vi "Get All Matched Nodes.vi"(8 "error in (no error)":errorcluster, 10 "XPath expression":string, 11 "node in":refnum<k20>) -> (0 "error out":errorcluster, 2 "node result array":refnum<k20>[](array[refnum]), 3 "node out":refnum<k20>)   [LabVIEW 2020, in "NI_XML.lvlib"]
doc: "Returns all the nodes within <B>node in</B> that match the <B>XPath expression</B>."
uses:
  <vilib>/xml/NI_XML.lvlib
  DOMUserDefRef.dll
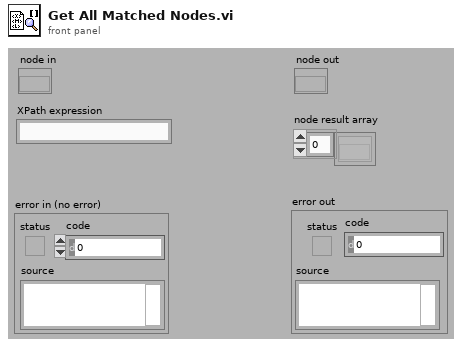
[diagram p1: front panel]
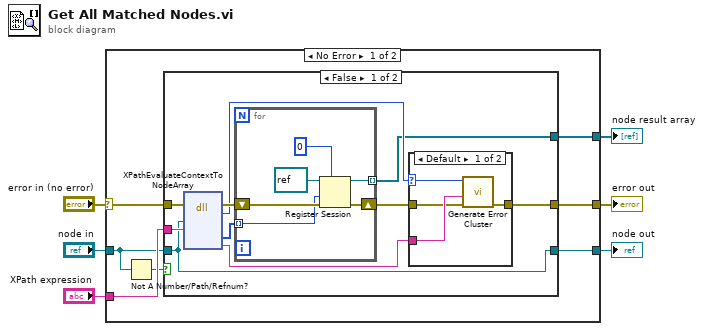
[diagram p0: block diagram]
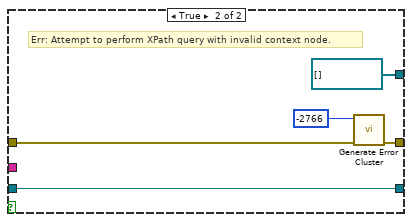
[diagram p3: hidden frame]
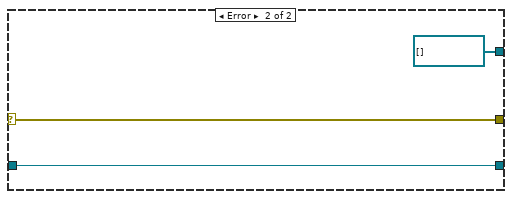
[diagram p4: hidden frame]
diagram:
  n1 = case shown="No Error" "error in (no error)" {
    selector: "error in (no error)" -> [w7 w42]
    tunnel: "XPath expression" -> [w13 _]
    tunnel: [w12 w42] -> w5
    tunnel: [w11 refnum<k20>[] []] -> w4
    tunnel: [w10 w41] -> w3
    tunnel: "node in" -> [w8 w41]
    frame No Error {
      n2 = Not A Number/Path/Refnum?(number/path/refnum=w8) -> (NaN/Path/Refnum?=w9:bool)
      n3 = case shown="False" w9 {
        tunnel: w13 -> [w23 _]
        tunnel: w7 -> [w20 w37]
        tunnel: w8 -> [w15 w39]
        tunnel: [w14 w36] -> w12
        tunnel: [w16 refnum<k20>[] []] -> w11
        tunnel: [w15 w39] -> w10
        frame False {
          n4 = dll-call lib="DOMUserDefRef.*" fn="XPathEvaluateContextToNodeArray"(error in=w20, "session"=w15, "xpathStr"=w23) -> (error out=w22:errorcluster, "retErr"=w18:i32, "retSess"=w21:u64[], "errIOString"=w19:string)  [unwired: 3 in, 4 out]
          n5 = for {
            tunnel: w21 -> [w30] mode=indexing
            tunnel: [w29] -> w16 mode=indexing
            shift-right: [w33] -> w17
            shift-left: w22 -> [w32]
            n6 = Register Session(7:0 ("cleanup mode (default to class = 0)"), 8:w32, 9:w30, 11:refnum<k20> refnum ("Node Reg")) -> (0:w33:errorcluster, 3:w29:refnum<k20>)  [unwired: 1 in]
          }
          n7 = case shown="Default" w18 {
            selector: w18 -> [w27 _]
            tunnel: w19 -> [w26 _]
            tunnel: w17 -> [w25 w28]
            tunnel: [w24 w28] -> w14
            frame Default {
              n8 = call <vilib>:"Generate Error Cluster.vi"("error in (no error)"=w25, "Additional Message"=w26, "Code"=w27) -> ("error out"=w24:errorcluster)  [unwired: 8 out]
            }
            frame 0 {
              # "No Error"
            }
          }
        }
        frame True {
          # "Err: Attempt to perform XPath query with invalid context node."
          n9 = call <vilib>:"Generate Error Cluster.vi"("error in (no error)"=w37, "Code"=-2766) -> ("error out"=w36:errorcluster)  [unwired: 1 in, 8 out]
        }
      }
    }
    frame Error {
    }
  }
  "error out" <- w5
  "node out" <- w3
  "node result array" <- w4
